vi "Stop Core.vi"(10 "final error code":i32, 11 "Base UI Actor in":refnum<class "Base UI Actor.lvclass">) -> (3 "Base UI Actor out":refnum<class "Base UI Actor.lvclass">)   [LabVIEW 2020, in "Base UI Actor.lvlib" / "Base UI Actor.lvclass"]
doc: "(<B>Filename</B>: Actor Framework.lvlib:Actor.lvclass:Stop Core.vi)\n\nDefines what the actor does before it stops. Use the <B>final error code</B> input to determine whether the actor shut down in response to an error.\n\nBy default, this method passes the Stop message along to all auto-stop nested actors. A descendant class may override this method to define additional behavior, such as shutting down any processes the actor initiated in its override of the Actor Core method."
uses:
  <vilib>/ActorFramework/Actor/Actor.lvclass/Actor.ctl
  <vilib>/ActorFramework/Stop Msg/Stop Msg.lvclass/Stop Msg.ctl
  <vilib>/ActorFramework/Message Enqueuer/Message Enqueuer.lvclass/Message Enqueuer.ctl
  <vilib>/ActorFramework/Stop Msg/Send Emergency Stop.vi
  <vilib>/ActorFramework/Stop Msg/Send Normal Stop.vi
  <vilib>/ActorFramework/Message Enqueuer/Enqueue Critical.vi
  <vilib>/ActorFramework/Message Enqueuer/Enqueue.vi
  <vilib>/ActorFramework/Stop Msg/Stop Msg.lvclass
  e:/builds/penguin/labview/branches/2020/dev/dist/vi.lib/ActorFramework/Message/Message.lvclass
  <vilib>/ActorFramework/Message Priority Queue/Priority Enqueue.vi
  Base UI Actor.lvclass
  <vilib>/ActorFramework/Actor/Actor.lvclass
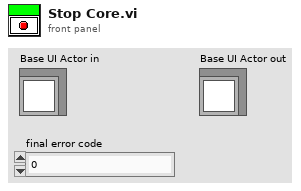
[diagram p1: front panel]
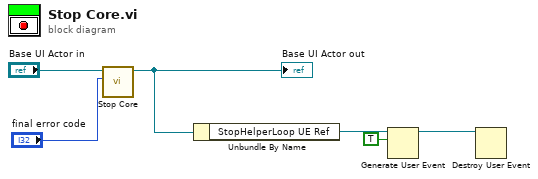
[diagram p0: block diagram]
diagram:
  n1 = call-parent "Stop Core.vi"("final error code"="final error code", "Actor in"="Base UI Actor in") -> ("Actor out"=w4:refnum<class "Base UI Actor.lvclass">)  [unwired: 9 in]
  "Base UI Actor out" <- w4
  n2 = Unbundle By Name(w4) -> ("StopHelperLoop UE Ref"=w3:refnum<user-event>)
  n3 = Generate User Event(user event=w3, event data cluster=TRUE ("event data")) -> (user event out=w1:refnum<user-event>)  [unwired: 2 in, 1 out]
  n4 = Destroy User Event(user event=w1) -> ()  [unwired: 1 in, 1 out]
